vi "Load ADC Table.vi"(1 "Error In":errorcluster) -> (0 "Error Out":errorcluster)   [LabVIEW 2018]
uses:
  Type Defs/RT Command.ctl
  Type Defs/Global Action.ctl
  <vilib>/Utility/config.llb/Write Key (String).vi
  <vilib>/Utility/config.llb/NI_LVConfig.lvlib
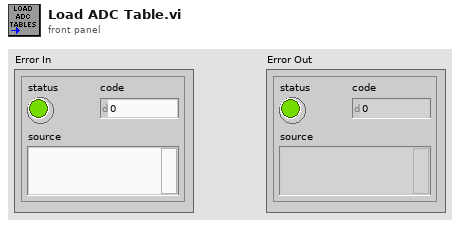
[diagram p1: front panel]
types:
  T1 = typedef "Global Action.ctl" = enum16{"Write", "Read"}
  T2 = typedef "RT Command.ctl" = enum16{"xml Start Run", "xml Start Actual Run", "xml Stop Run", "xml Runtime Update", "xml Get Status", "xml Get Table", "xml Set Table", "xml Get Configuration", "xml System Status", "xml Set LC Input Logic", "xml Get Data", "xml Get Info", "Start", "StartActualRun", "Stop", "Runtime Update", "Get Data", "Get Info", "Get Status", "Get Param", "Get Config", "Get Table", "Read ADC", "Set Oscillator", "Update Config", "Update Table", "Set All Pol", "Set Pol and DC", "Set Max Mass", "Toggle RP", "Toggle EL", "Set PIC", "Initialize Turbo", "Send Turbo Comm", "Close Turbo", "P1", "P2", "P3", "Send Serial", "Set LC Out", "Get LC In", "Read VAC", "Test Table", "Toggle Power", "Get Startup", "Set Startup", "Get ADC Table", "Set ADC Table", "Get Brief Status", "Get Detail Status", "Auxiliary Update", "Set CC Logics", "Set CC Input Logics", "Ignore Error", "invalid"}
  T3 = typedef "Global Configrations.ctl" = cluster{"Model Name":enum16{"QSight 110", "QSight 120", "QSight 210", "QSight 220", "QSight 410", "QSight 420", "IONICS 3Q 110", "IONICS 3Q 120", "IONICS 3Q 210", "IONICS 3Q 220", "IONICS 3Q 310", "IONICS 3Q 320", "Simulation (Single Source)", "Simulation (Dual Source)"}, "RunType":u16, "Acquisition State":enum16{"Ready", "Busy", "Waiting"}, "InstrState":enum16{"Initializing", "Mass Spectrometer is Off", "Starting Up", "Turning Power Off", "Going to Standby", "Roughing Pump Ready", "Turning Turbo Off", "Turbo Startup", "Turbopump Ready", "Checking Vacuum", "Going to Ready", "Ready", "Running", "Source Standby", "Lost Communication", "Shutting Down", "Fault", "24V Standby", "Go to 24V Standby", "Turbopump Ready-Waiting"}, "Run Mode":enum16{"MRM (Q1/Q2)", "Q1 Scan", "Q1 SRM", "Q2 Scan", "Q2 SRM", "Product Scan", "Precursor Scan", "Neutral Loss", "Neutral Gain"}, "Configration":T4, "TCP ID":refnum<k5>, "DT":bool, "Dead Time (nS)":i32, "Single Source":bool, "ADC Tables":T6[], "FW Udate":bool, "Simulator":bool}
  T4 = typedef "Configration.ctl" = cluster{"Table":T5[], "Instrument":string[]}
  T5 = typedef "Function Lib.lvlib/_RT Configuration 2.ctl" = cluster{"Name":string, "Ch#":u8, "Min":dbl, "Max":dbl, "Def+":dbl, "Def-":dbl, "Offset":dbl, "Slope":dbl, "Type":u8, "Description":string, "SettleT":dbl}
  T6 = typedef "ADC Table.ctl" = cluster{"Name":string, "Ch#":u8, "Min":dbl, "Max":dbl, "Def+":dbl, "Def-":dbl, "Offset":dbl, "Slope":dbl, "Type":u8, "Description":string, "SettleT":dbl}
  T7 = typedef "NI_LVConfig.lvlib/Config Data RefNum.ctl" = refnum<k1>
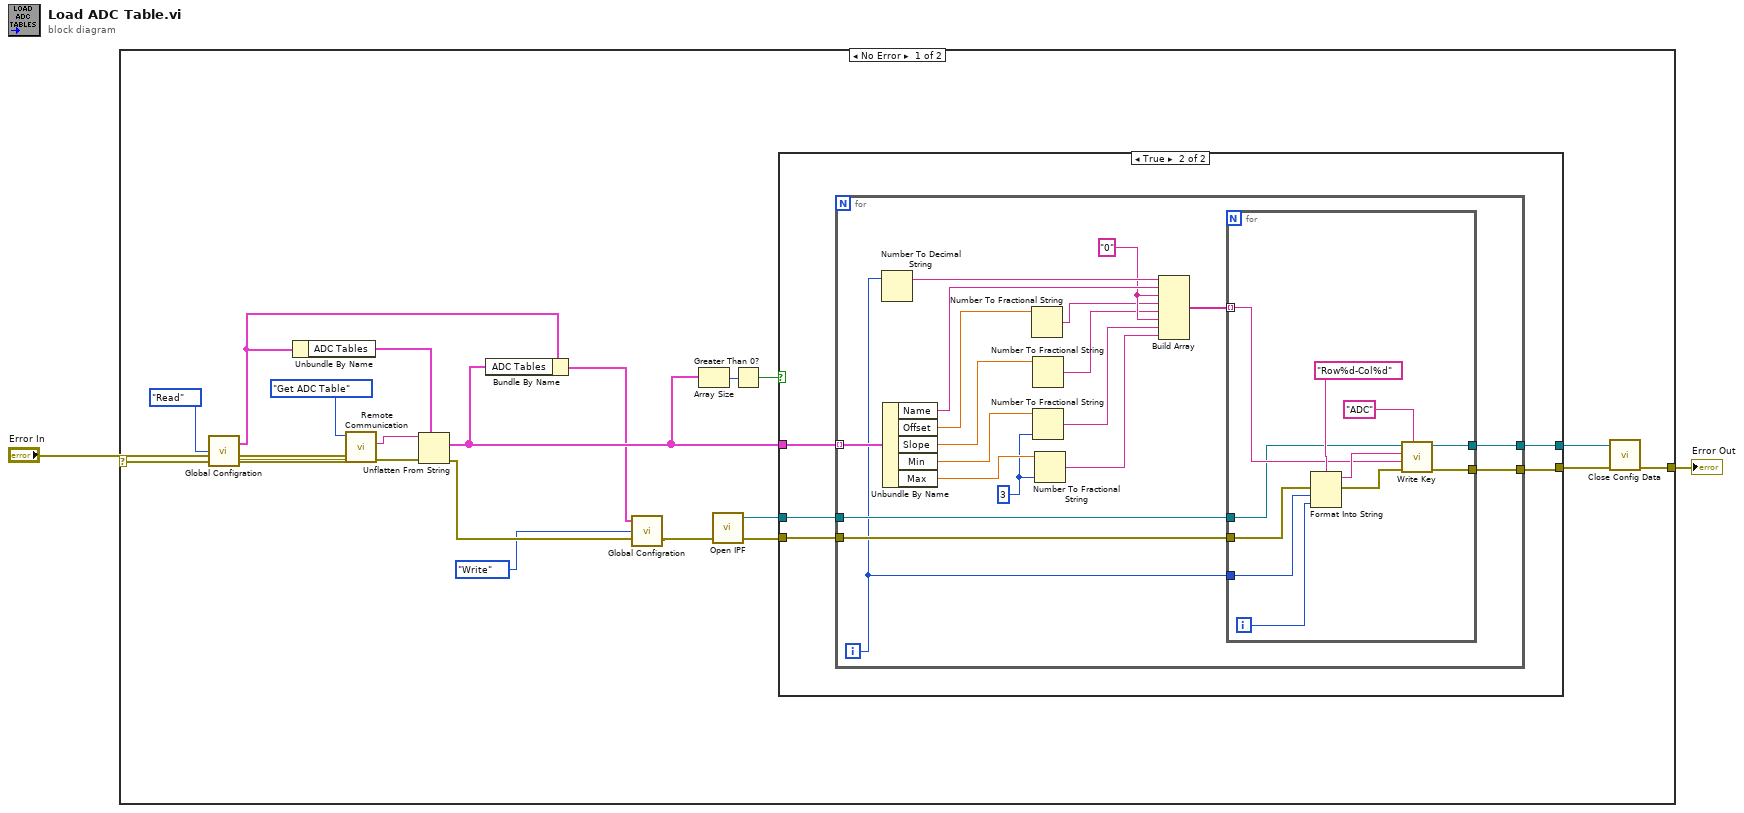
[diagram p0: block diagram]
diagram:
  n1 = case shown="No Error" "Error In" {
    selector: "Error In" -> [w11 w60]
    tunnel: [w13 w60] -> w1
    frame No Error {
      n2 = call "Global Configration.vi"("Error In"=w11, "Action"=Global_Action."Read") -> ("Error Out"=w12:errorcluster, "Parameters Out"=w5:T3)  [unwired: 1 in]
      n3 = Unbundle By Name(w5) -> ("ADC Tables"=w9:T6[])
      n4 = call "Remote Communication.vi"("Error In"=w12, "Command"=RT_Command."Get ADC Table") -> ("Error Out"=w20:errorcluster, "Info"=w19:string)  [unwired: 4 in, 2 out]
      n5 = Unflatten From String(type=w9, binary string=w19, error in (no error)=w20) -> (value=w4:T6[], error out=w8:errorcluster)  [unwired: 3 out]
      n6 = Bundle By Name(cluster=w5, "ADC Tables"=w4) -> (w3:T3)
      n7 = call "Global Configration.vi"("Error In"=w8, "Action"=Global_Action."Write", "Parameters In"=w3) -> ("Error Out"=w7:errorcluster)  [unwired: 1 out]
      n8 = Array Size(array=w4) -> (size(s)=w21:i32)
      n9 = call "Open IPF.vi"("Error In"=w7) -> ("Error Out"=w17:errorcluster, "IPF refnum"=w16:T7)  [unwired: 2 in, 1 out]
      n10 = Greater Than 0?(x=w21) -> (x > 0?=w18:bool)
      n11 = case shown="True" w18 {
        tunnel: w17 -> [w24 w27]
        tunnel: w16 -> [w23 w28]
        tunnel: w4 -> [_ w29]
        tunnel: [w23 w26] -> w15
        tunnel: [w24 w25] -> w14
        frame False {
        }
        frame True {
          n12 = for {
            tunnel: w29 -> [w48] mode=indexing
            tunnel: w28 -> [w34]
            tunnel: w27 -> [w35]
            tunnel: [w31] -> w26
            tunnel: [w30] -> w25
            i -> [w32]
            w36 = i16 3 ("precision (6)")
            w44 = "0"
            n13 = Number To Decimal String(number=w32) -> (decimal integer string=w47:string)  [unwired: 1 out]
            n14 = Unbundle By Name(w48) -> ("Name"=w46:string, "Offset"=w45:dbl, "Slope"=w42:dbl, "Min"=w41:dbl, "Max"=w40:dbl)
            n15 = Number To Fractional String(number=w45) -> (F-format string=w43:string)  [unwired: 3 out]
            n16 = Number To Fractional String(number=w42) -> (F-format string=w39:string)  [unwired: 3 out]
            n17 = Number To Fractional String(number=w41, precision (6)=w36) -> (F-format string=w38:string)  [unwired: 2 out]
            n18 = Number To Fractional String(number=w40, precision (6)=w36) -> (F-format string=w37:string)  [unwired: 2 out]
            n19 = Build Array(w47, w46, w44, w43, w39, w44, w38, w37) -> (w33:string[])
            n20 = for {
              tunnel: w35 -> [w54]
              tunnel: w34 -> [w55]
              tunnel: w33 -> [w56] mode=indexing
              tunnel: w32 -> [w53]
              tunnel: [w50] -> w31
              tunnel: [w49] -> w30
              i -> [w52]
              n21 = Format Into String(format string="Row%d-Col%d" ("section"), error in=w54, w53, w52) -> (resulting string=w58:string, error out=w51:errorcluster)  [unwired: 1 in]
              n22 = call-poly <vilib>:"Write Key.vi"("section"="ADC", "error in (no error)"=w51, "value"=w56, "key"=w58, "refnum"=w55) -> ("error out"=w49:errorcluster, "refnum out"=w50:T7)  [unwired: 1 in, 4 out]
            }
          }
        }
      }
      n23 = call <vilib>:"Close Config Data.vi"("error in (no error)"=w14, "refnum"=w15) -> ("error out"=w13:errorcluster)  [unwired: 1 in, 8 out]
    }
    frame Error {
    }
  }
  "Error Out" <- w1
